vi "Hide.vi"(0 "reference in":refnum<class "DataGridView.lvclass">, 11 "error in (no error)":errorcluster) -> (4 "reference out":refnum<class "DataGridView.lvclass">, 15 "error out":errorcluster)   [LabVIEW 2018, in "DataGridView.lvclass"]
doc: "Hides the DataGridView"
uses:
  DataGridView.lvclass
  System.Windows.Forms
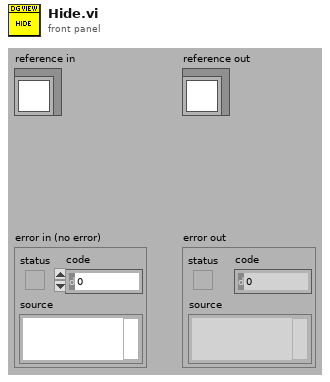
[diagram p1: front panel]
types:
  T1 = typedef "DataGridView.lvclass/ObjectAttributes.ctl" = cluster{"DataGridView":refnum<k24>, "SelectionChangedEvent":refnum<user-event>, "SelectionChanged callback ref":refnum<k27>, "LastSelectedRowIndex":i32}
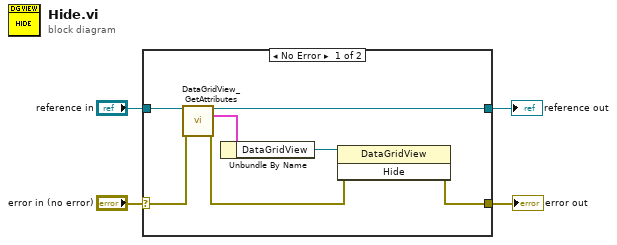
[diagram p0: block diagram]
diagram:
  n1 = case shown="No Error" "error in (no error)" {
    selector: "error in (no error)" -> [w11 w13]
    tunnel: [w5 w13] -> w3
    tunnel: [w8 w12] -> w1
    tunnel: "reference in" -> [w9 w12]
    frame No Error {
      n2 = call "DataGridView_GetAttributes.vi"("reference in"=w9, "error in (no error)"=w11) -> ("reference out"=w8:refnum<class "DataGridView.lvclass">, "Data"=w10:T1, "error out"=w6:errorcluster)  [unwired: 10 in, 1 out]
      n3 = Unbundle By Name(w10) -> ("DataGridView"=w7:refnum<k24>)
      n4 = invoke class="DataGridView" method="Hide"(reference=w7, error in=w6) -> (error out=w5:errorcluster)  [unwired: 1 in, 2 out]
    }
    frame Error {
    }
  }
  "error out" <- w3
  "reference out" <- w1
